vi "CRYGet Graph Control by Legend.vi"(0 "Graph Type":string, 5 "DataView Index":i32, 7 "Graph Number":i32) -> (2 "Display Number":i32, 3 "Graph VI Ref":refnum<vi>, 4 "Wave Graph Ref":refnum<vi>, 6 "XY Graph Ref":refnum<vi>, 8 "Digital Graph Ref":refnum<vi>, 10 "Bar Graph Ref":refnum<vi>, 12 "Table GMListbox Ref":refnum<vi>, 13 "Result GMListbox Ref":refnum<vi>, 14 "Text Graph Ref":refnum<vi>, 15 "Polar/Picture Graph Ref":refnum<vi>)   [LabVIEW 2013]
uses:
  CRYData View Global.vi
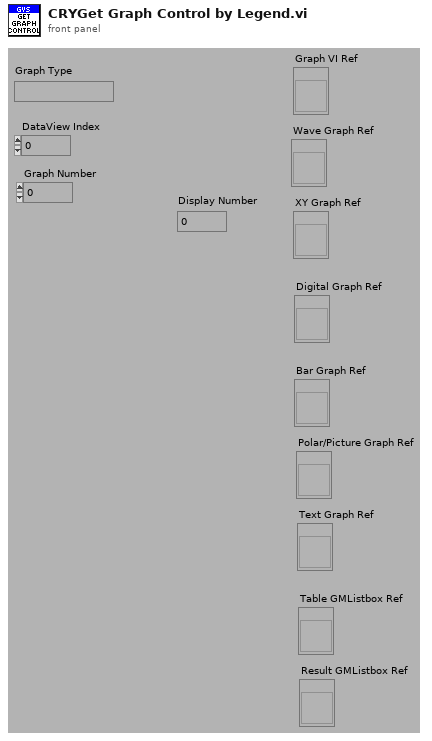
[diagram p1: front panel]
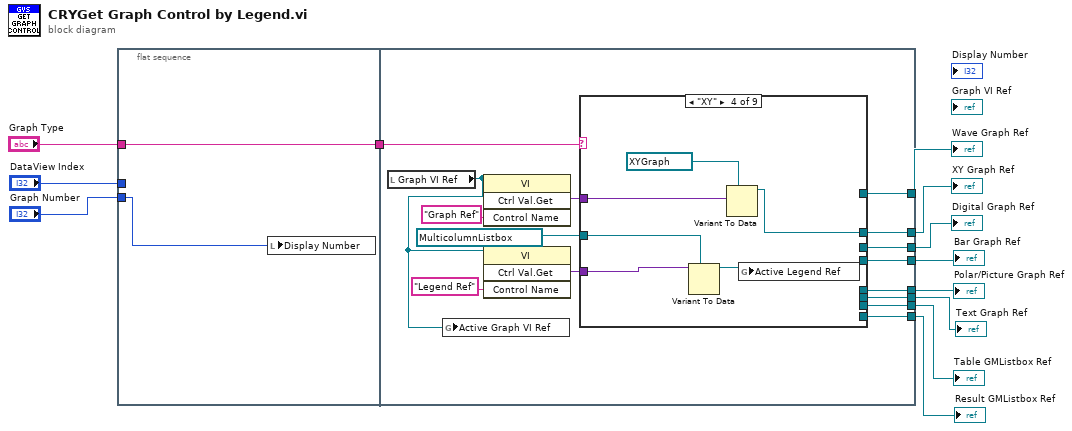
[diagram p0: block diagram]
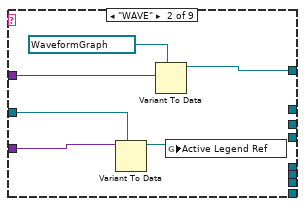
[diagram p3: hidden frame]
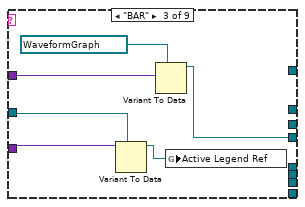
[diagram p4: hidden frame]
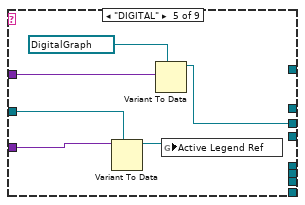
[diagram p5: hidden frame]
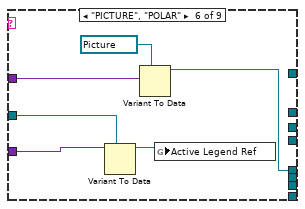
[diagram p6: hidden frame]
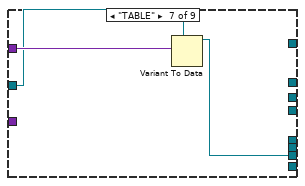
[diagram p7: hidden frame]
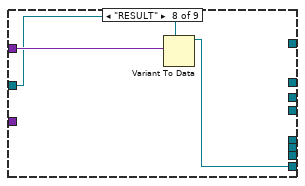
[diagram p8: hidden frame]
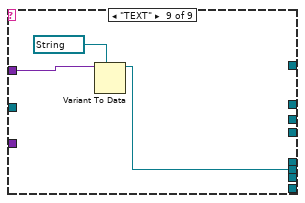
[diagram p9: hidden frame]
diagram:
  n1 = flat-sequence {
    tunnel: "DataView Index" -> [_]
    tunnel: "Graph Number" -> [w13]
    tunnel: [w14] -> w3
    tunnel: "Graph Type" -> [w14]
    tunnel: [w29] -> w12
    tunnel: [w28] -> w11
    tunnel: [w27] -> w10
    tunnel: [w26] -> w9
    tunnel: [w25] -> w8
    tunnel: [w24] -> w7
    tunnel: [w23] -> w6
    tunnel: w3 -> [w17]
    tunnel: [w15] -> w1
    frame #0 {
      n2 = local write "Display Number"(w13) -> ()
    }
    frame #1 {
      n3 = local read "Graph VI Ref"() -> (w18:refnum<vi>)
      n4 = global write "CRYData View Global.vi" "Active Graph VI Ref"(w18) -> ()
      n5 = invoke class="VI" method="Ctrl Val.Get"(reference=w18, "Control Name"="Graph Ref") -> ("Get Control Value Variant"=w22:variant)  [unwired: 2 in, 3 out]
      n6 = invoke class="VI" method="Ctrl Val.Get"(reference=w18, "Control Name"="Legend Ref") -> ("Get Control Value Variant"=w19:variant)  [unwired: 2 in, 3 out]
      n7 = case shown="\"XY\"" w17 {
        tunnel: [_ w35 _ _ _ _ _ _ _] -> w29
        tunnel: w22 -> [_ w34 w41 w47 w53 w59 w62 w65 w67]
        tunnel: [_ _ _ w45 _ _ _ _ _] -> w28
        tunnel: [_ _ _ _ w52 _ _ _ _] -> w27
        tunnel: [_ _ w39 _ _ _ _ _ _] -> w26
        tunnel: w19 -> [_ w31 w37 w43 w50 w55 _ _ _]
        tunnel: [_ _ _ _ _ _ w61 _ _] -> w24
        tunnel: [_ _ _ _ _ w57 _ _ _] -> w25
        tunnel: [_ _ _ _ _ _ _ w64 _] -> w23
        tunnel: refnum<vi> refnum ("Legend Ref") -> [_ w30 w36 w42 w48 w54 w60 w63 _]
        tunnel: [_ _ _ _ _ _ _ _ w66] -> w15
        frame "False", Default {
        }
        frame "WAVE" {
          n8 = Variant To Data(type=w30, Variant=w31) -> (data=w32:refnum<vi>)  [unwired: 1 in, 1 out]
          n9 = Variant To Data(type=refnum<vi> refnum ("WaveGraph Ref"), Variant=w34) -> (data=w35:refnum<vi>)  [unwired: 1 in, 1 out]
          n10 = global write "CRYData View Global.vi" "Active Legend Ref"(w32) -> ()
        }
        frame "BAR" {
          n11 = Variant To Data(type=w36, Variant=w37) -> (data=w38:refnum<vi>)  [unwired: 1 in, 1 out]
          n12 = Variant To Data(type=refnum<vi> refnum ("WaveGraph Ref"), Variant=w41) -> (data=w39:refnum<vi>)  [unwired: 1 in, 1 out]
          n13 = global write "CRYData View Global.vi" "Active Legend Ref"(w38) -> ()
        }
        frame "XY" {
          n14 = Variant To Data(type=w42, Variant=w43) -> (data=w44:refnum<vi>)  [unwired: 1 in, 1 out]
          n15 = Variant To Data(type=refnum<vi> refnum ("XY Graph"), Variant=w47) -> (data=w45:refnum<vi>)  [unwired: 1 in, 1 out]
          n16 = global write "CRYData View Global.vi" "Active Legend Ref"(w44) -> ()
        }
        frame "DIGITAL" {
          n17 = Variant To Data(type=w48, Variant=w50) -> (data=w49:refnum<vi>)  [unwired: 1 in, 1 out]
          n18 = Variant To Data(type=refnum<vi> refnum ("Graph Ref"), Variant=w53) -> (data=w52:refnum<vi>)  [unwired: 1 in, 1 out]
          n19 = global write "CRYData View Global.vi" "Active Legend Ref"(w49) -> ()
        }
        frame "PICTURE", "POLAR" {
          n20 = Variant To Data(type=w54, Variant=w55) -> (data=w56:refnum<vi>)  [unwired: 1 in, 1 out]
          n21 = Variant To Data(type=refnum<vi> refnum ("Graph Ref"), Variant=w59) -> (data=w57:refnum<vi>)  [unwired: 1 in, 1 out]
          n22 = global write "CRYData View Global.vi" "Active Legend Ref"(w56) -> ()
        }
        frame "TABLE" {
          n23 = Variant To Data(type=w60, Variant=w62) -> (data=w61:refnum<vi>)  [unwired: 1 in, 1 out]
        }
        frame "RESULT" {
          n24 = Variant To Data(type=w63, Variant=w65) -> (data=w64:refnum<vi>)  [unwired: 1 in, 1 out]
        }
        frame "TEXT" {
          n25 = Variant To Data(type=refnum<vi> refnum ("WaveGraph Ref"), Variant=w67) -> (data=w66:refnum<vi>)  [unwired: 1 in, 1 out]
        }
      }
    }
  }
  "XY Graph Ref" <- w11
  "Wave Graph Ref" <- w12
  "Digital Graph Ref" <- w10
  "Bar Graph Ref" <- w9
  "Polar/Picture Graph Ref" <- w8
  "Table GMListbox Ref" <- w7
  "Result GMListbox Ref" <- w6
  "Text Graph Ref" <- w1
